vi "Principal01.vi"() -> ()   [LabVIEW 2012]
panel:
  out "Sinal":bool
  out "POSI敲O":dbl(graph)
  in  "Porta Serial":refnum<visa-resource-name>="COM7"
  in  "?":bool
  out "Read String":string
  in  "Write String":string="*IDN?\r\n"
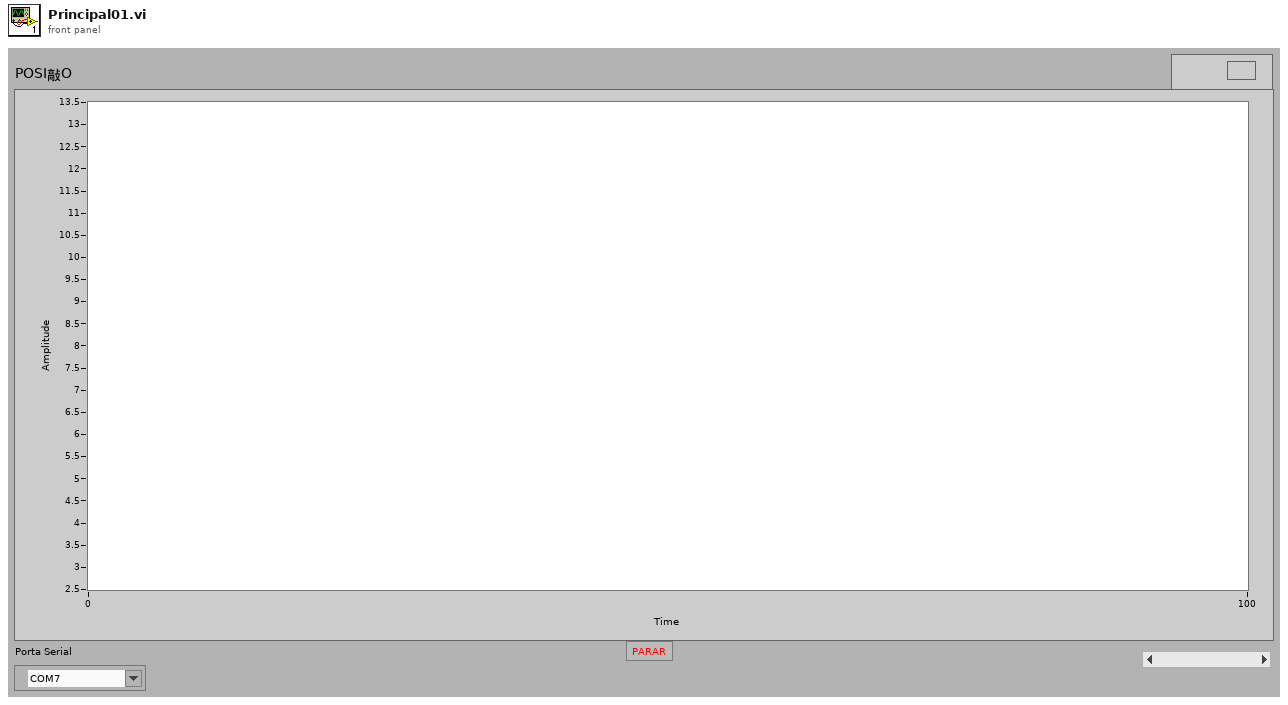
[diagram p1: front panel]
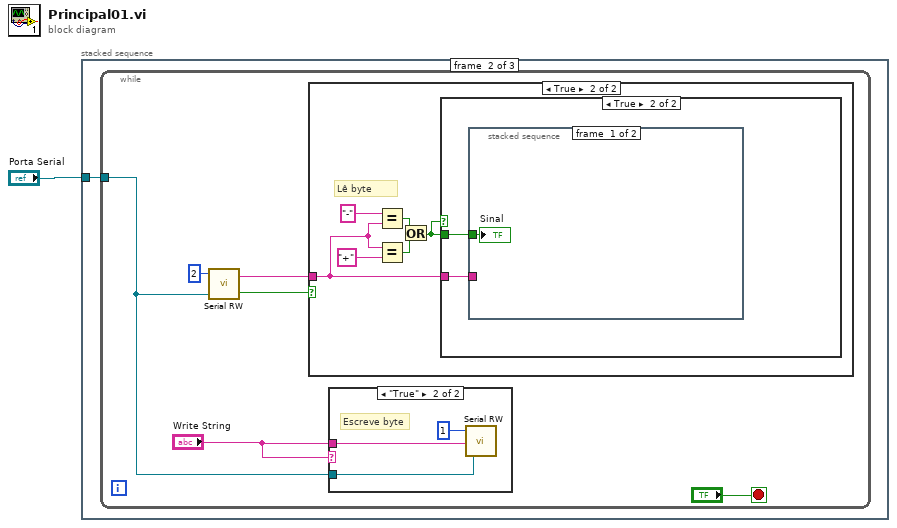
[diagram p0: block diagram]
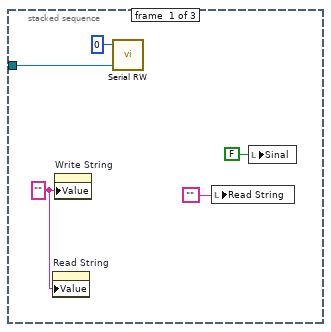
[diagram p2: hidden frame]
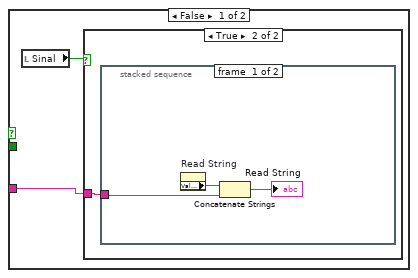
[diagram p5: hidden frame]
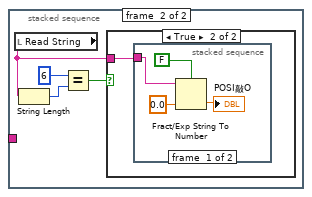
[diagram p7: hidden frame]
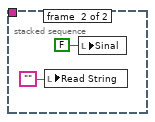
[diagram p9: hidden frame]
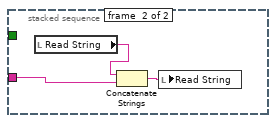
[diagram p10: hidden frame]
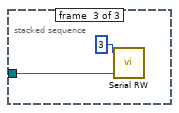
[diagram p11: hidden frame]
diagram:
  n1 = stacked-sequence {
    tunnel: "Porta Serial" -> [w4 w7 w46]
    frame #0 {
      w6 = "" ("string to write")
      n2 = property on="Read String" class="Str"("Value"=w6) -> ()  [unwired: 2 in, 2 out]
      n3 = property on="Write String" class="Str"("Value"=w6) -> ()  [unwired: 2 in, 2 out]
      n4 = call "Serial RW.vi"("Porta Serial"=w4, "Função"=u8 0) -> ()  [unwired: 1 in, 2 out]
      n5 = local write "Read String"("") -> ()
      n6 = local write "Sinal"(FALSE ("Sinal")) -> ()
    }
    frame #1 {
      n7 = while {
        tunnel: w7 -> [w10]
        stop <- "?" stop-if-true
        n8 = call "Serial RW.vi"("Porta Serial"=w10, "Função"=u8 2) -> ("TemDado"=w12:bool, "Leitura"=w8:string)  [unwired: 1 in]
        n9 = case shown="True" w12 {
          tunnel: w8 -> [_ w18]
          frame False {
          }
          frame True {
            # "Lê byte"
            n10 = Equal?(x="-", y=w18) -> (x = y?=w22:bool)
            n11 = Equal?(x=w18, y="+") -> (x = y?=w21:bool)
            n12 = Or(x=w22, y=w21) -> (x .or. y?=w17:bool)
            n13 = case shown="True" w17 {
              tunnel: w17 -> [_ w41]
              tunnel: w18 -> [w23 w40]
              frame False {
                n14 = local read "Sinal"() -> (w24:bool)
                n15 = case shown="True" w24 {
                  tunnel: w23 -> [_ w25]
                  frame False {
                  }
                  frame True {
                    n16 = stacked-sequence {
                      tunnel: w25 -> [w28 _]
                      frame #0 {
                        n17 = property on="Read String" class="Str"() -> ("Value"=w27:string)  [unwired: 2 in, 2 out]
                        n18 = Concatenate Strings(w27, w28) -> (→"Read String":string)
                      }
                      frame #1 {
                        n19 = local read "Read String"() -> (w30:string)
                        n20 = String Length(string=w30) -> (length=w32:i32)
                        n21 = Equal?(x=6 ("y"), y=w32) -> (x = y?=w29:bool)
                        n22 = case shown="True" w29 {
                          tunnel: w30 -> [_ w33]
                          frame False {
                          }
                          frame True {
                            n23 = stacked-sequence {
                              tunnel: w33 -> [w36 _]
                              frame #0 {
                                n24 = Fract/Exp String To Number(use system decimal point (T)=FALSE, string=w36, default (0 dbl)=0.0 ("default (0 DBL)")) -> (number=→"POSI敲O":dbl)  [unwired: 1 in, 1 out]
                              }
                              frame #1 {
                                n25 = local write "Read String"("") -> ()
                                n26 = local write "Sinal"(FALSE ("Sinal")) -> ()
                              }
                            }
                          }
                        }
                      }
                    }
                  }
                }
              }
              frame True {
                n27 = stacked-sequence {
                  tunnel: w41 -> [w42 _]
                  tunnel: w40 -> [_ w45]
                  frame #0 {
                    "Sinal" <- w42
                  }
                  frame #1 {
                    n28 = local read "Read String"() -> (w43:string)
                    n29 = Concatenate Strings(w43, w45) -> (w44:string)
                    n30 = local write "Read String"(w44) -> ()
                  }
                }
              }
            }
          }
        }
        n31 = case shown="\"True\"" "Write String" {
          tunnel: "Write String" -> [_ w15]
          tunnel: w10 -> [_ w14]
          frame "False", Default {
          }
          frame "True" {
            # "Escreve byte"
            n32 = call "Serial RW.vi"("Porta Serial"=w14, "Escrita"=w15, "Função"=u8 1) -> ()  [unwired: 2 out]
          }
        }
      }
    }
    frame #2 {
      n33 = call "Serial RW.vi"("Porta Serial"=w46, "Função"=u8 3) -> ()  [unwired: 1 in, 2 out]
    }
  }
